vi "Write TriggerEdge.vi"(8 "error in (no error)":errorcluster, 10 "TriggerEdge":T1, 11 "T560Trigger in":refnum<class "T560Trigger.lvclass">) -> (0 "error out":errorcluster, 3 "T560Trigger out":refnum<class "T560Trigger.lvclass">)   [LabVIEW 2013, in "Highlandt564.lvlib" / "T560Trigger.lvclass"]
uses:
  T560Trigger.lvclass
  Common/TypeDefs/TiggerEdge.ctl
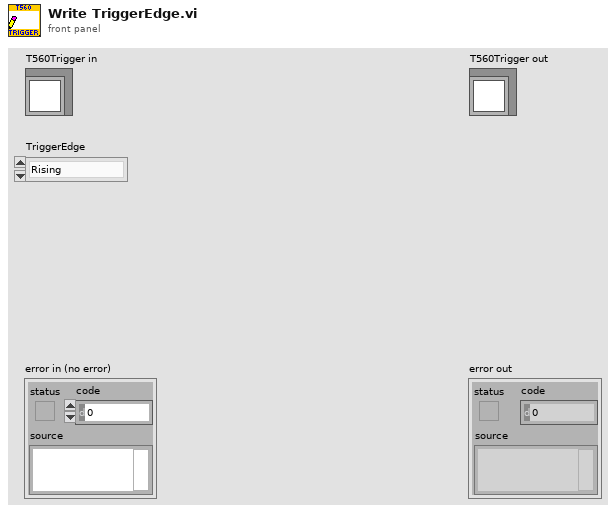
[diagram p1: front panel]
types:
  T1 = typedef "TiggerEdge.ctl" = enum16{"Rising", "Falling"}
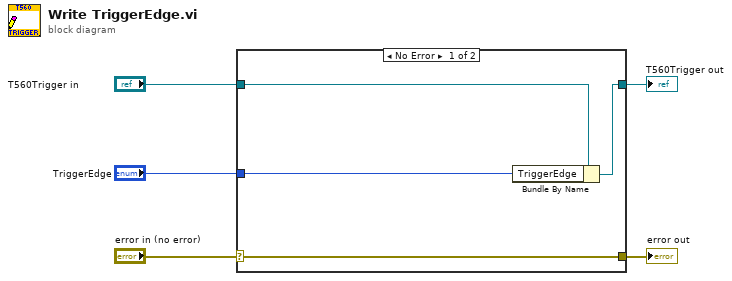
[diagram p0: block diagram]
diagram:
  n1 = case shown="No Error" "error in (no error)" {
    selector: "error in (no error)" -> [w9 w10]
    tunnel: [w9 w10] -> w4
    tunnel: [w7 w11] -> w2
    tunnel: "T560Trigger in" -> [w8 w11]
    tunnel: "TriggerEdge" -> [w6 _]
    frame No Error {
      n2 = Bundle By Name(cluster=w8, "TriggerEdge"=w6) -> (w7:refnum<class "T560Trigger.lvclass">)
    }
    frame Error {
    }
  }
  "error out" <- w4
  "T560Trigger out" <- w2
